vi "Get Message-Enqueuer-References Type Information.vi"(8 "error in (no error)":errorcluster, 11 "Message Enqueuer References":path) -> (0 "error out":errorcluster, 3 "Event Ref Information":T1[](array[typedef]))   [LabVIEW 2018, in "Scripting.lvlib"]
uses:
  Scripting.lvlib
  Event-Type-Information.ctl
  Error-Codes.ctl
  Error-Offset.vi
  <vilib>/Utility/error.llb/Error Cluster From Error Code.vi
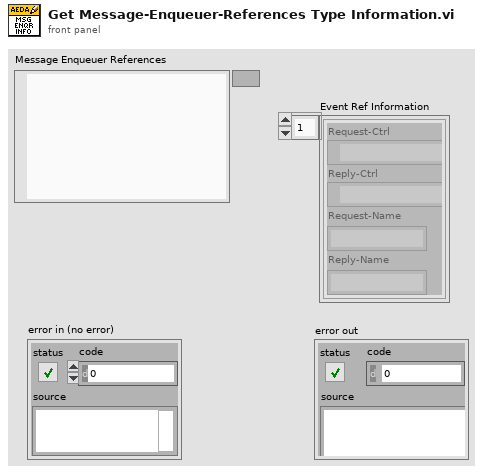
[diagram p1: front panel]
types:
  T1 = typedef "Scripting.lvlib/Event-Type-Information.ctl" = cluster{"Request-Ctrl":path, "Reply-Ctrl":path, "Request-Name":string, "Reply-Name":string}
  T2 = typedef "Scripting.lvlib/Error-Codes.ctl" = enum16{"EVENT_REF_TYPE_DEF_IS_NESTED", "EVENT_REF_TYPE_DEF_IS_EMPTY", "EVENT_REF_TYPE_DEF_INCLUDES_NON_REFS", "EVENT_REF_TYPE_INVALID_REPLY_REF", "EVENT_REF_TYPE_REPLY_IS_NOT_TYPE_DEF", "EVENT_REF_TYPE_DEF_IS_NOT_CLUSTER", "EVENT_REF_TYPE_DEF_INVALID_REQ_REPLY_TYPE", "ACTOR_CLASS_PATH_IS_INVALID", "ACTOR_CLASS_LIBRARY_IS_NOT_EDITABLE", "ACTOR_CLASS_CREATE_ENQUEUER_REFS_VI_NOT_FOUND", "MSG_ENQUEUER_REFS_CTL_NOT_FOUND", "ACTOR_CLASS_MAIN_RUN_VI_NOT_FOUND", "ACTOR_CLASS_DESTROY_ENQUEUER_REFS_VI_NOT_FOUND", "CREATE_ENQUEUER_REFS_ERROR_TERMINAL_NOT_FOUND", "CREATE_ENQUEUER_REFS_INVALID_TYPE_DEF", "CREATE_ENQUEUER_REF_NAMEBUNDLER_NOT_FOUND", "CREATE_ENQUEUER_REF_MULTIPLE_NAMEBUNDLERS", "MESSAGES_REF_TYPE_DEF_IS_EMPTY", "MESSAGES_REF_TYPE_DEF_IS_NESTED", "ACTOR_TEMPLATE_CLASS_NOT_FOUND"}
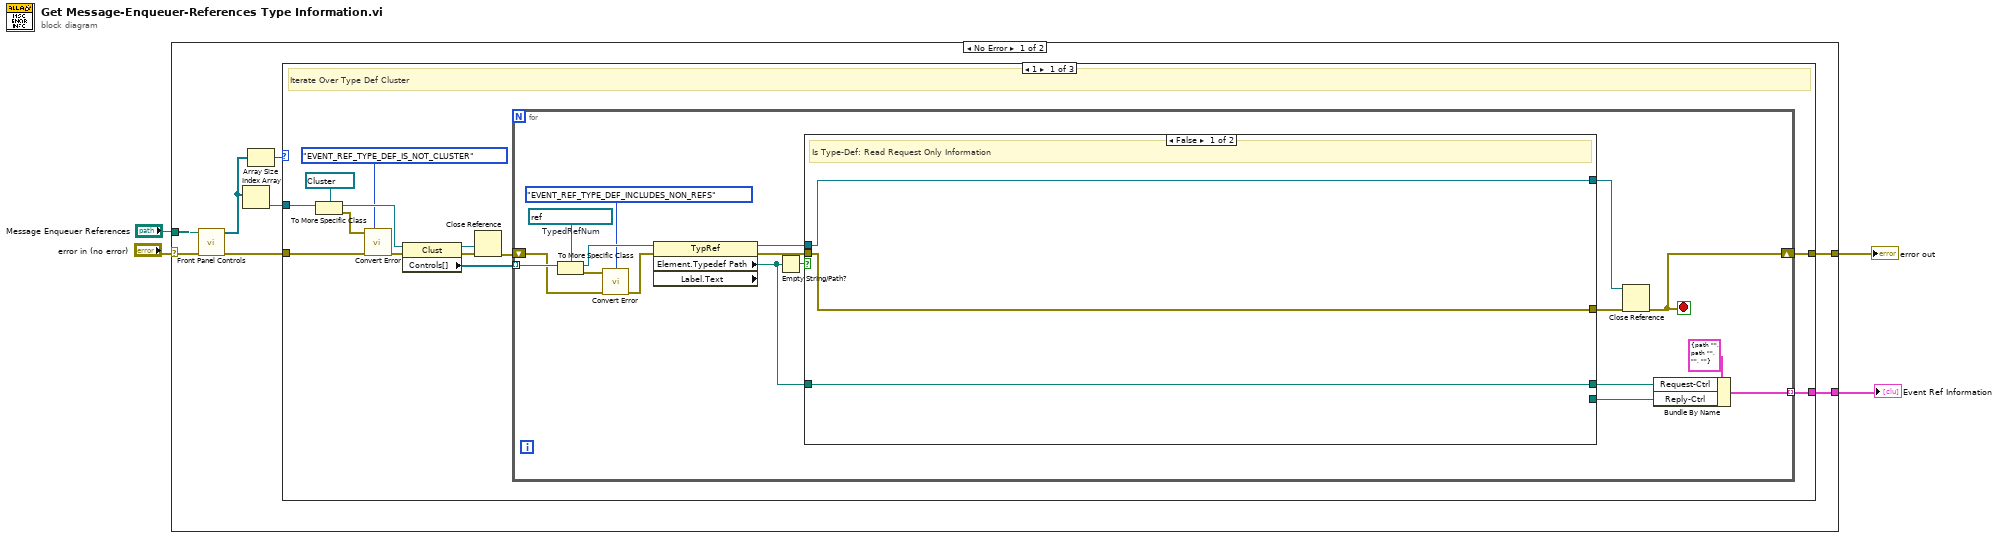
[diagram p0: block diagram]
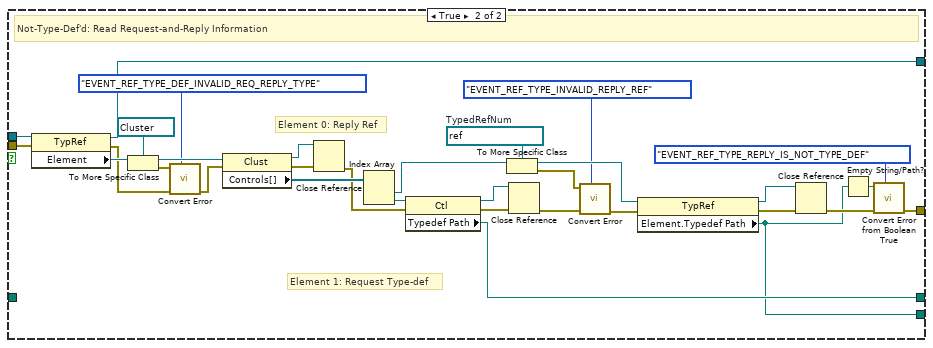
[diagram p2: hidden frame]
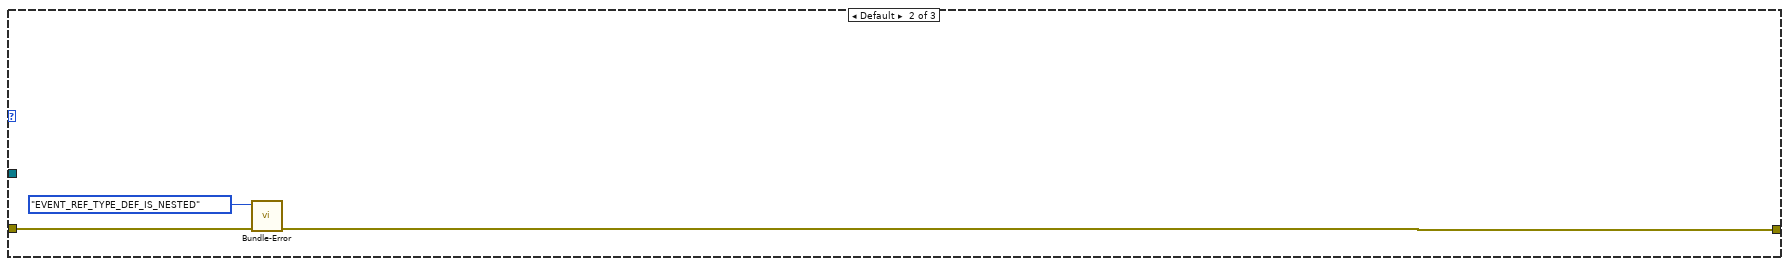
[diagram p3: hidden frame]
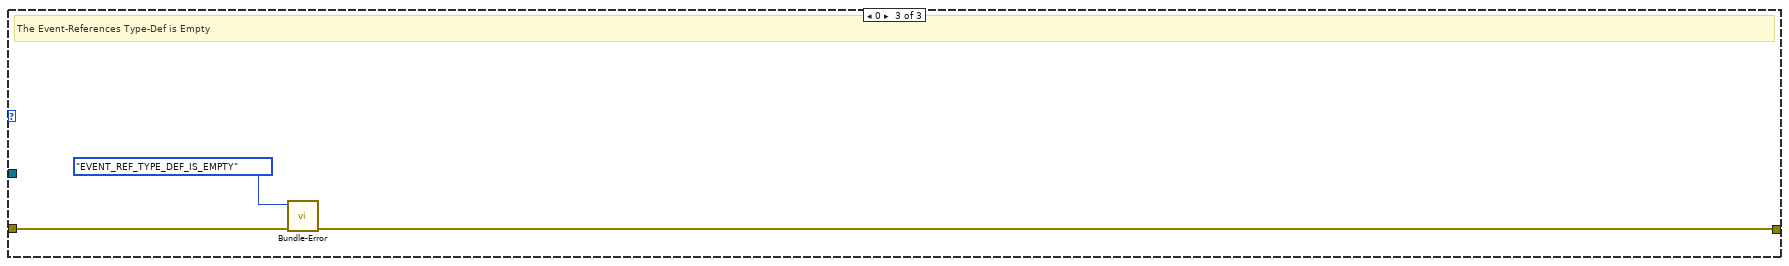
[diagram p4: hidden frame]
diagram:
  n1 = case shown="No Error" "error in (no error)" {
    selector: "error in (no error)" -> [w11 w85]
    tunnel: "Message Enqueuer References" -> [w12 _]
    tunnel: [w8 _] -> w2
    tunnel: [w5 w85] -> w1
    frame No Error {
      n2 = call "Front Panel Controls.vi"("error in (no error)"=w11, "VI/Type-Def Path"=w12) -> ("error out"=w6:errorcluster, "Controls[]"=w9:refnum<vi>[])  [unwired: 8 in]
      n3 = Index Array(array=w9) -> (element=w7:refnum<vi>)  [unwired: 1 in]
      n4 = Array Size(array=w9) -> (size(s)=w10:i32)
      n5 = case shown="1" w10 {
        tunnel: [w24 w81 w83] -> w5
        tunnel: w7 -> [w21 _ _]
        tunnel: [w23 _ _] -> w8
        tunnel: w6 -> [w18 w79 w82]
        frame 1 {
          # "Iterate Over Type Def Cluster"
          n6 = To More Specific Class(target class=refnum<vi> refnum ("Type"), reference=w21) -> (specific class reference=w20:refnum<vi>, error out=w17:errorcluster)  [unwired: 1 in]
          n7 = call "Convert Error.vi"("Convert to Error Code"=Error-Codes."EVENT_REF_TYPE_DEF_IS_NOT_CLUSTER" ("Errors"), "error in (no error)"=w18, "Error Input"=w17) -> ("error out"=w19:errorcluster)  [unwired: 8 in]
          n8 = property class="Clust"(reference=w20, error in=w19) -> (reference out=w13:refnum<vi>, error out=w14:errorcluster, "Controls[]"=w25:refnum<vi>[])
          n9 = Close Reference(reference=w13, error in (no error)=w14) -> (error out=w15:errorcluster)
          n10 = for {
            tunnel: w25 -> [w43] mode=indexing
            shift-right: [w26] -> w24
            shift-left: w15 -> [w34]
            tunnel: [w41] -> w23 mode=indexing
            stop <- w26 stop-if-true
            w32 = refnum<vi> refnum  # TypedRefNum
            n11 = To More Specific Class(target class=w32, reference=w43) -> (specific class reference=w42:refnum<vi>, error out=w35:errorcluster)  [unwired: 1 in]
            n12 = call "Convert Error.vi"("Convert to Error Code"=Error-Codes."EVENT_REF_TYPE_DEF_INCLUDES_NON_REFS" ("Errors"), "error in (no error)"=w34, "Error Input"=w35) -> ("error out"=w33:errorcluster)  [unwired: 8 in]
            n13 = property class="TypRef" props=["Element", "Typedef Path", "Label", "Text"](reference=w42, error in=w33) -> (reference out=w39:refnum<vi>, error out=w38:errorcluster, "Element.Typedef Path"=w37:path)  [unwired: 1 out]
            n14 = Empty String/Path?(string/path=w37) -> (empty?=w40:bool)
            n15 = case shown="False" w40 {
              tunnel: w39 -> [w45 w78]
              tunnel: w38 -> [w44 w77]
              tunnel: [w44 w51] -> w27
              tunnel: [w46 w72] -> w30
              tunnel: [_ w50] -> w29
              tunnel: w37 -> [w46 _]
              tunnel: [w45 w47] -> w28
              frame False {
                # "Is Type-Def: Read Request Only Information"
              }
              frame True {
                w65 = refnum<vi> refnum  # TypedRefNum
                # "Element 1: Request Type-def"
                # "Element 0: Reply Ref"
                # "Not-Type-Def'd: Read Request-and-Reply Information"
                n16 = property class="TypRef"(reference=w78, error in=w77) -> (reference out=w47:refnum<vi>, error out=w48:errorcluster, "Element"=w76:refnum<vi>)
                n17 = To More Specific Class(target class=refnum<vi> refnum ("Type"), reference=w76) -> (specific class reference=w75:refnum<vi>, error out=w55:errorcluster)  [unwired: 1 in]
                n18 = call "Convert Error.vi"("Convert to Error Code"=Error-Codes."EVENT_REF_TYPE_DEF_INVALID_REQ_REPLY_TYPE" ("Errors"), "error in (no error)"=w48, "Error Input"=w55) -> ("error out"=w56:errorcluster)  [unwired: 8 in]
                n19 = property class="Clust"(reference=w75, error in=w56) -> (reference out=w68:refnum<vi>, error out=w69:errorcluster, "Controls[]"=w70:refnum<vi>[])
                n20 = Close Reference(reference=w68, error in (no error)=w69) -> (error out=w67:errorcluster)
                n21 = Index Array(array=w70) -> (element #1=w61:refnum<vi>, element #2=w66:refnum<vi>)  [unwired: 2 in]
                n22 = property class="Ctl"(reference=w66, error in=w67) -> (reference out=w73:refnum<vi>, error out=w74:errorcluster, "Typedef Path"=w72:path)
                n23 = To More Specific Class(target class=w65, reference=w61) -> (specific class reference=w64:refnum<vi>, error out=w58:errorcluster)  [unwired: 1 in]
                n24 = Close Reference(reference=w73, error in (no error)=w74) -> (error out=w60:errorcluster)
                n25 = call "Convert Error.vi"("Convert to Error Code"=Error-Codes."EVENT_REF_TYPE_INVALID_REPLY_REF" ("Errors"), "error in (no error)"=w60, "Error Input"=w58) -> ("error out"=w59:errorcluster)  [unwired: 8 in]
                n26 = property class="TypRef"(reference=w64, error in=w59) -> (reference out=w63:refnum<vi>, error out=w62:errorcluster, "Element.Typedef Path"=w50:path)
                n27 = Close Reference(reference=w63, error in (no error)=w62) -> (error out=w53:errorcluster)
                n28 = Empty String/Path?(string/path=w50) -> (empty?=w49:bool)
                n29 = call "Convert Error from Boolean True.vi"("Convert to Error Code"=Error-Codes."EVENT_REF_TYPE_REPLY_IS_NOT_TYPE_DEF" ("Errors"), "error in (no error)"=w53, "Error Input"=w49) -> ("error out"=w51:errorcluster)  [unwired: 8 in]
              }
            }
            n30 = Close Reference(reference=w28, error in (no error)=w27) -> (error out=w26:errorcluster)
            n31 = Bundle By Name(cluster=T1 {"Request-Ctrl"=path "", "Reply-Ctrl"=path "", "Request-Name"="", "Reply-Name"=""} ("output cluster"), "Request-Ctrl"=w30, "Reply-Ctrl"=w29) -> (w41:T1)
          }
        }
        frame Default {
          n32 = call "Bundle-Error.vi"("error in (no error)"=w79, "Errors"=Error-Codes."EVENT_REF_TYPE_DEF_IS_NESTED") -> ("error out"=w81:errorcluster)  [unwired: 9 in]
        }
        frame 0 {
          # "The Event-References Type-Def is Empty"
          n33 = call "Bundle-Error.vi"("error in (no error)"=w82, "Errors"=Error-Codes."EVENT_REF_TYPE_DEF_IS_EMPTY") -> ("error out"=w83:errorcluster)  [unwired: 9 in]
        }
      }
    }
    frame Error {
    }
  }
  "Event Ref Information" <- w2
  "error out" <- w1
